vi "Detector Abort FG.vi"(7 "init":bool, 8 "error in (no error)":errorcluster, 11 "state":bool) -> (0 "error out":errorcluster, 3 "abort?":bool)   [LabVIEW 2022 SP3, in "PRIME Detector.lvclass"]
uses:
  PRIME Detector.lvclass
  PRIME Detector.lvclass/PRIME Detector.ctl
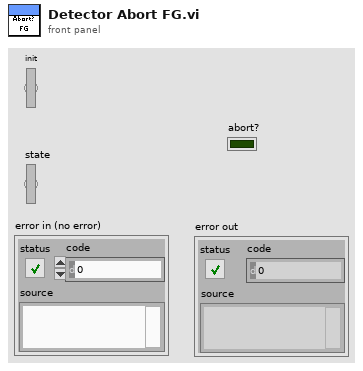
[diagram p1: front panel]
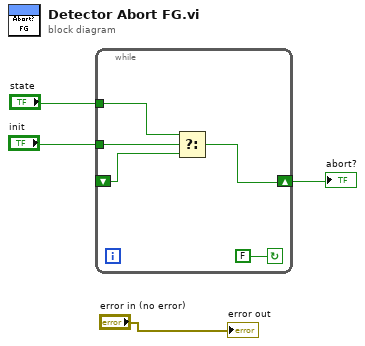
[diagram p0: block diagram]
diagram:
  n1 = while {
    shift-right: [w7] -> w2
    shift-left: _ -> [w6]
    tunnel: "init" -> [w9]
    tunnel: "state" -> [w8]
    stop <- FALSE continue-if-true
    n2 = Select(t=w8, s=w9, f=w6) -> (s? t:f=w7:bool)
  }
  "abort?" <- w2
  "error out" <- "error in (no error)"
